vi "kCounterI64.vi"(10 "Reset":bool) -> (1 "Dynamic Counter":i64, 3 "Static Counter":i64)   [LabVIEW 2010, in "KevLib01.lvlib"]
uses:
  KevLib01.lvlib
panel:
  # "Counter:\n\nIncrements every loop iteration.  It freezes the counter and transfers it to static Counter when ever reset it high.\n\nWARNING: DOES NOT LIKE TWO CONSECUTIVE RESETS"
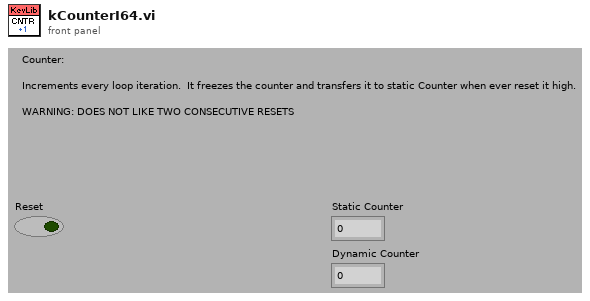
[diagram p1: front panel]
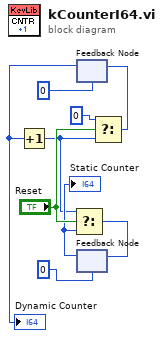
[diagram p0: block diagram]
diagram:
  n1 = feedback #1(i64 0) -> (w7:i64)
  "Dynamic Counter" <- w7
  n2 = Increment(x=w7) -> (x+1=w3:i64)
  n3 = feedback #2(i64 0 ("f")) -> (w8:i64)
  "Static Counter" <- w8
  n4 = Select(t=w3, s="Reset", f=w8) -> (s? t:f=w5:i64)
  n5 = feedback-in #2(w5) -> ()
  n6 = Select(t=i64 0 ("f"), s="Reset", f=w3) -> (s? t:f=w1:i64)
  n7 = feedback-in #1(w1) -> ()
